vi "Handle Relative Path.vi"(8 "error in (no error)":errorcluster, 10 "Path":path) -> (0 "error out":errorcluster, 2 "appended path":path)   [LabVIEW 2020, in "LUnitCLI.lvclass"]
uses:
  LUnitCLI.lvclass
  LUnitCLI.lvclass/LUnitCLI.ctl
  kernel32.dll
  libc.so.6
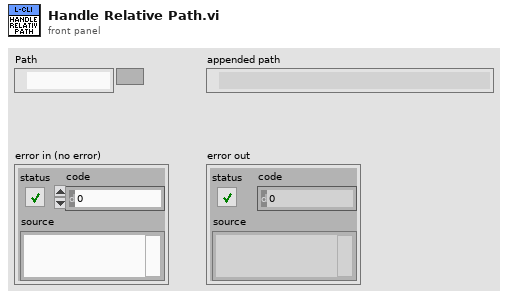
[diagram p1: front panel]
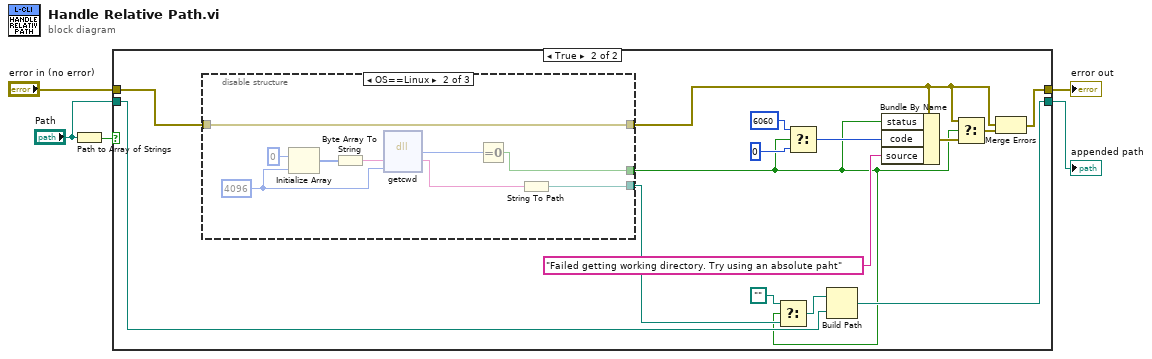
[diagram p0: block diagram]
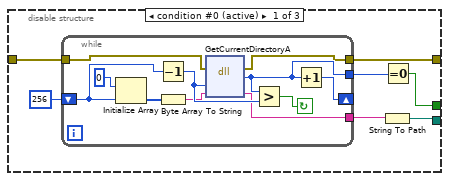
[diagram p3: hidden frame]
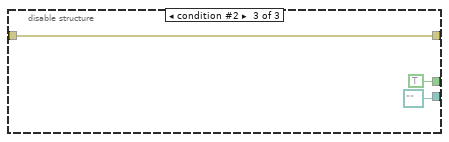
[diagram p4: hidden frame]
diagram:
  n1 = Path to Array of Strings(0:"Path") -> (1:w3:bool)  [unwired: 1 out]
  n2 = case shown="True" w3 {
    tunnel: [w6 w20] -> w1
    tunnel: "error in (no error)" -> [w6 w19]
    tunnel: "Path" -> [w7 w22]
    tunnel: [w7 w21] -> w5
    frame False {
    }
    frame True {
      n3 = disable-structure shown="OS==Linux" {
        disable-tunnel: w19 -> [w29 w49 w52]
        disable-tunnel: [w28 w49 w52] -> w17
        disable-tunnel: [w25 w41 path ""] -> w9
        disable-tunnel: [w23 w43 TRUE] -> w8
        frame condition #0 (active) {
          n4 = while {
            tunnel: [w37] -> w24
            tunnel: [w34] -> w26
            shift-left: 256 -> [w40]
            shift-right: [w38] -> _
            tunnel: w29 -> [w31]
            tunnel: [w30] -> w28
            stop <- w39 continue-if-true
            n5 = Initialize Array(u8 0 ("U8"), w40) -> (w33:u8[])
            n6 = Decrement(x=w40) -> (x-1=w36:i32)
            n7 = Byte Array To String(unsigned byte array=w33) -> (string=w35:string)
            n8 = dll-call lib="kernel32.dll" fn="GetCurrentDirectoryA"(error in=w31, "buflen"=w36, "szDir"=w35) -> (error out=w30:errorcluster, w37:i32, "szDir"=w34:string)  [unwired: 3 in, 1 out]
            n9 = Greater?(x=w37, y=w36) -> (0:w39:bool)
            n10 = Increment(x=w37) -> (x+1=w38:i32)
          }
          n11 = String To Path(string=w26) -> (path=w25:path)
          n12 = Equal To 0?(x=w24) -> (x = 0?=w23:bool)
        }
        frame condition #1 {
          w45 = u64 4096 ("element")
          n13 = Initialize Array(u8 0 ("element"), w45) -> (w47:u8[])
          n14 = Byte Array To String(unsigned byte array=w47) -> (string=w46:string)
          n15 = dll-call lib="libc.so.6" fn="getcwd"("buf"=w46, "size"=w45) -> ("return type"=w44:u64, "buf"=w42:string)  [unwired: 4 in, 2 out]
          n16 = Equal To 0?(x=w44) -> (x = 0?=w43:bool)
          n17 = String To Path(string=w42) -> (path=w41:path)
        }
        frame condition #2 {
        }
      }
      n18 = Select(t=path "", s=w8, f=w9) -> (s? t:f=w18:path)
      n19 = Select(t=6060, s=w8, f=0) -> (s? t:f=w12:i32)
      n20 = Build Path(base path=w18, name or relative path=w22) -> (appended path=w21:path)
      n21 = Bundle By Name(cluster=w17, "status"=w8, "code"=w12, "source"="Failed getting working directory. Try using an absolute paht") -> (w11:errorcluster)
      n22 = Select(t=w17, s=w8, f=w11) -> (s? t:f=w16:errorcluster)
      n23 = Merge Errors(w17, w16) -> (w20:errorcluster)
    }
  }
  "appended path" <- w5
  "error out" <- w1
